vi "NI VeriStand - Get Item Path.vi"(8 "error in (no error)":errorcluster, 11 "Item Ref in":T1 format="%.0x") -> (0 "error out":errorcluster, 2 "Path":string, 3 "Item Ref out":T1 format="%.0x", 4 "Found":bool)   [LabVIEW 2020, in "Custom Device API.lvlib"]
doc: "Returns the System Explorer path to the custom device item specified by <B>Item Ref in</B>."
uses:
  <vilib>/NI VeriStand/Custom Device API/Custom Device API.lvlib
  <vilib>/NI VeriStand/Custom Device API/Custom Device Item Ref.ctl
  1279fc91-3ca6-45af-aadb-8a851be273cb.vi
  <vilib>/NI VeriStand/Custom Device API/Custom Device Offline Path.vi
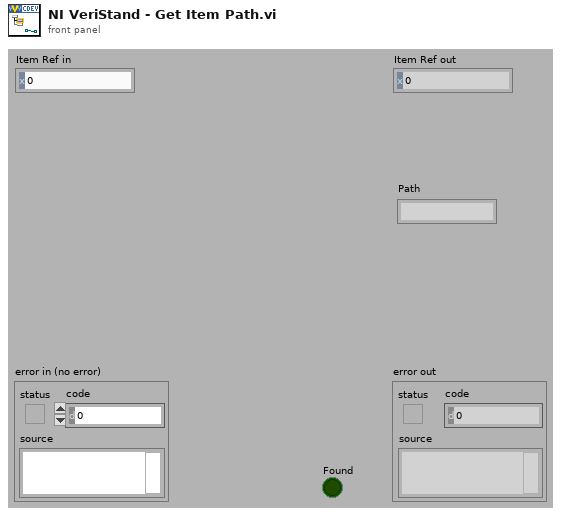
[diagram p1: front panel]
types:
  T1 = typedef "Custom Device API.lvlib/Custom Device Item Ref.ctl" = u64
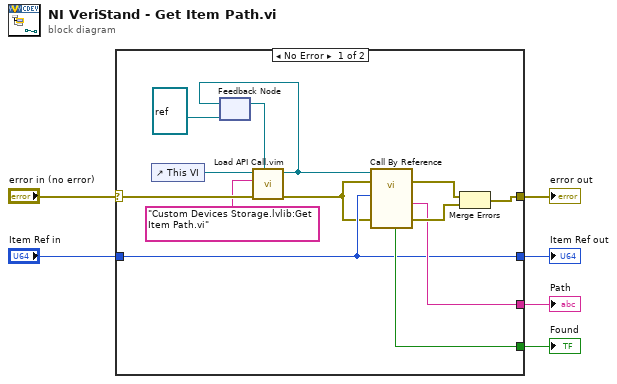
[diagram p0: block diagram]
diagram:
  n1 = case shown="No Error" "error in (no error)" {
    selector: "error in (no error)" -> [w12 w21]
    tunnel: [w18 w21] -> w6
    tunnel: "Item Ref in" -> [w15 w20]
    tunnel: [w15 w20] -> w4
    tunnel: [w17 _] -> w3
    tunnel: [w16 _] -> w2
    frame No Error {
      n2 = control-ref of="This VI"() -> (w13:refnum<vi>)
      n3 = feedback #1(refnum<vi> refnum ("type specifier VI Refnum (for type only)")) -> (w14:refnum<vi>)
      n4 = call "Load API Call.vim"("VI reference in"=w14, "error in (no error)"=w12, "VI qualified name"="Custom Devices Storage.lvlib:Get Item Path.vi", "Caller VI ref"=w13) -> ("error out"=w11:errorcluster, "VI reference"=w10:refnum<vi>)  [unwired: 6 in]
      n5 = feedback-in #1(w10) -> ()
      n6 = call-by-ref "?"(reference=w10, error in=w11, 8:"error in (no error)"=w11, "Item Ref in"=w15) -> (error out=w7:errorcluster, 0:"error out"=w19:errorcluster, "Item Path"=w17:string, "Found"=w16:bool)  [unwired: 6 in, 2 out]
      n7 = Merge Errors(w7, w19) -> (w18:errorcluster)
    }
    frame Error {
    }
  }
  "Item Ref out" <- w4
  "error out" <- w6
  "Found" <- w2
  "Path" <- w3
